vi "data_rec_vi.vi"() -> ()   [LabVIEW 2019]
panel:
  out "token string 5":string
  out "token string 4":string
  out "token string 3":string
  out "token string 2":string
  out "token string":string
  out "data out":string
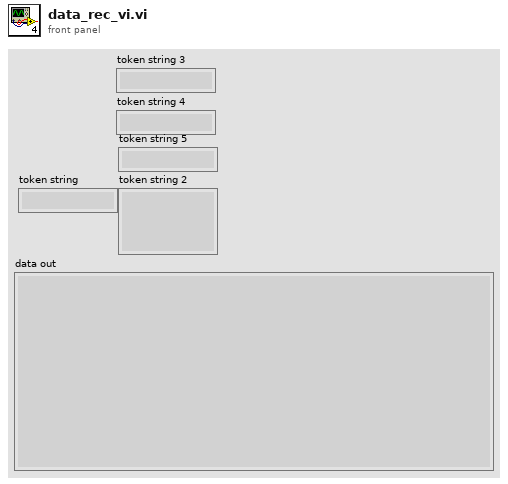
[diagram p1: front panel]
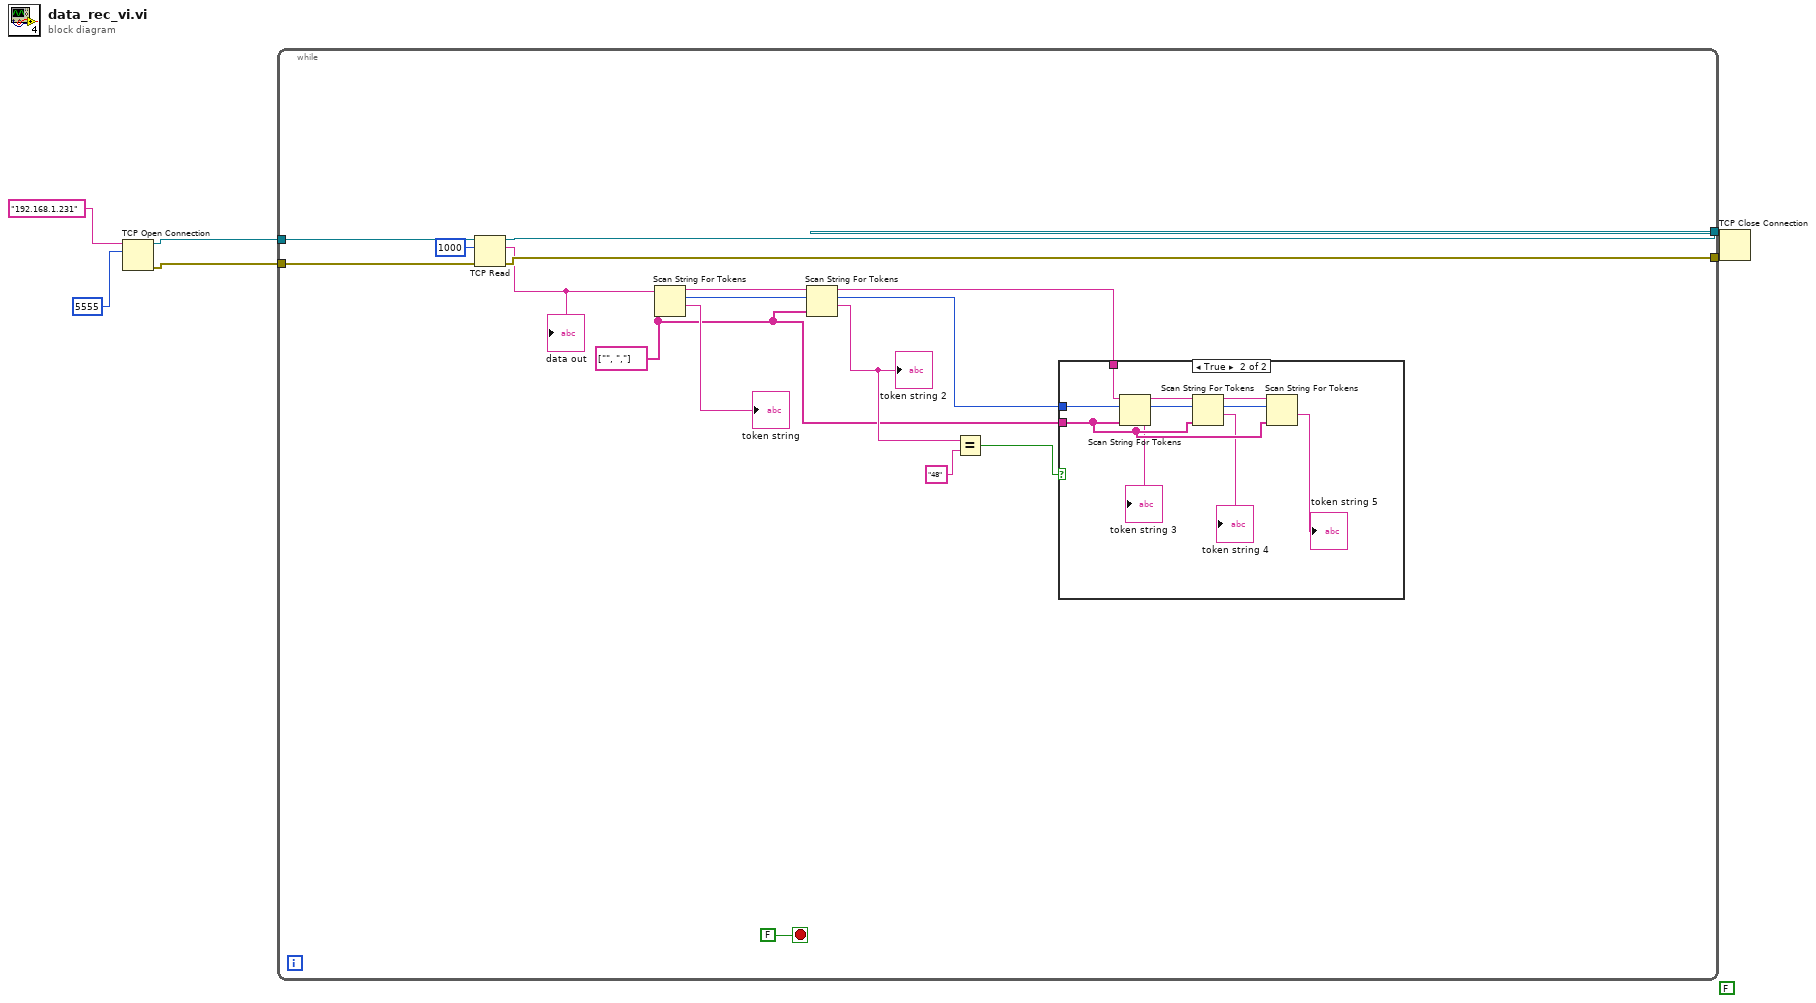
[diagram p0: block diagram]
diagram:
  (unwired) FALSE
  n1 = TCP Open Connection(address="192.168.1.231", remote port or service name=u16 5555) -> (connection ID=w6:refnum<k5>, error out=w4:errorcluster)  [unwired: 3 in]
  n2 = while {
    tunnel: w6 -> [w22]
    tunnel: [w21] -> w5
    tunnel: w4 -> [w20]
    tunnel: [w19] -> w3
    stop <- FALSE stop-if-true
    w7 = string[] ["", ","] ("delimiters (\\s,\\t,\\r,\\n)")
    n3 = TCP Read(connection ID=w22, bytes to read=1000, error in (no error)=w20) -> (connection ID out=w21:refnum<k5>, data out=w16:string, error out=w19:errorcluster)  [unwired: 2 in]
    "data out" <- w16
    n4 = Scan String For Tokens(6:w7, 9:w16) -> (1:→"token string":string, 2:w14:i32, 3:w13:string)  [unwired: 4 in, 1 out]
    n5 = Scan String For Tokens(6:w7, 8:w14, 9:w13) -> (1:w12:string, 2:w8:i32, 3:w9:string)  [unwired: 3 in, 1 out]
    "token string 2" <- w12
    n6 = Equal?(x=w12, y="48") -> (x = y?=w10:bool)
    n7 = case shown="True" w10 {
      tunnel: w9 -> [_ w28]
      tunnel: w8 -> [_ w27]
      tunnel: w7 -> [_ w26]
      frame False {
      }
      frame True {
        n8 = Scan String For Tokens(6:w26, 8:w27, 9:w28) -> (1:→"token string 3":string, 2:w30:i32, 3:w32:string)  [unwired: 3 in, 1 out]
        n9 = Scan String For Tokens(6:w26, 8:w30, 9:w32) -> (1:→"token string 4":string, 2:w29:i32, 3:w31:string)  [unwired: 3 in, 1 out]
        n10 = Scan String For Tokens(6:w26, 8:w29, 9:w31) -> (1:→"token string 5":string)  [unwired: 3 in, 3 out]
      }
    }
  }
  n11 = TCP Close Connection(connection ID=w5, error in (no error)=w3) -> ()  [unwired: 1 in, 2 out]
